vi "RemoveDuplicateChar.vi"(1 "Input String":string) -> (0 "Discrete String":string)   [LabVIEW 2015]
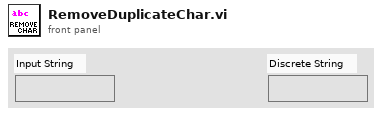
[diagram p1: front panel]
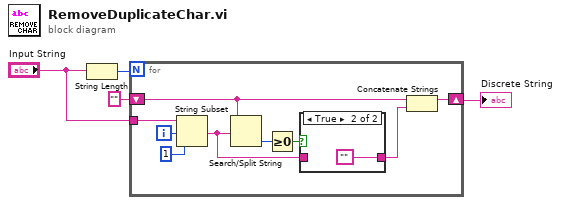
[diagram p0: block diagram]
diagram:
  n1 = String Length(string="Input String") -> (length=w4:i32)
  n2 = for {
    N: w4 -> [_]
    shift-right: [w10] -> w1
    shift-left: "" -> [w6]
    tunnel: "Input String" -> [w13]
    i -> [w11]
    n3 = String Subset(string=w13, offset (0)=w11, length (rest)=1 ("length (rest)")) -> (substring=w5:string)
    n4 = Search/Split String(string=w6, search string/char (-)=w5) -> (offset of match=w9:i32)  [unwired: 1 in, 2 out]
    n5 = Greater Or Equal To 0?(x=w9) -> (x >= 0?=w8:bool)
    n6 = case shown="True" w8 {
      tunnel: [w14 ""] -> w7
      tunnel: w5 -> [w14 _]
      frame False {
      }
      frame True {
      }
    }
    n7 = Concatenate Strings(w6, w7) -> (w10:string)
  }
  "Discrete String" <- w1
